vi "设置模块队列名.vi"() -> (3 "Msg":string)   [LabVIEW 2016, in "斯坦道CODMn.lvlib"]
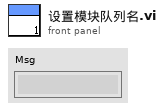
[diagram p1: front panel]
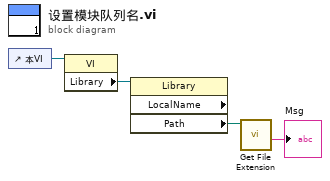
[diagram p0: block diagram]
diagram:
  n1 = control-ref of="本VI"() -> (w4:refnum<vi>)
  n2 = property class="VI"(reference=w4) -> ("Library"=w2:refnum<vi>)  [unwired: 1 in, 2 out]
  n3 = property class="Library" props=["LocalName", "Path"](reference=w2) -> ("Path"=w3:path)  [unwired: 1 in, 3 out]
  n4 = call <vilib>:"Get File Extension.vi"("file"=w3) -> ("filename without extension"=→"Msg":string)  [unwired: 6 in, 4 out]
